vi "Render Delimiter.vi"(8 "Error In":errorcluster) -> (0 "Error Out":errorcluster)   [LabVIEW 2018, in "Tests.lvlib" / "Render.lvlib"]
uses:
  Render.lvlib
  src/Toolkit/Data/Map/Map.lvclass
  D:/Users/cfield/Code/Field R&D Services/Mustache/LabVIEW/trunk/src/Toolkit/Data/Abstract/Abstract.lvclass
  src/Toolkit/Low-Level/Support/Lex String.vi
  src/Toolkit/Data/Map/Support/From String Array.vi
  src/Toolkit/Low-Level/Support/Render to String.vi
  <vilib>/addons/_JKI Toolkits/Caraya/classes/Test/Test.lvclass
  <vilib>/addons/_JKI Toolkits/Caraya/classes/Assert/Assert.lvclass
  src/Toolkit/Toolkit.lvlib
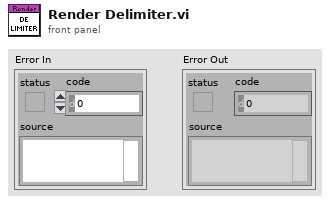
[diagram p1: front panel]
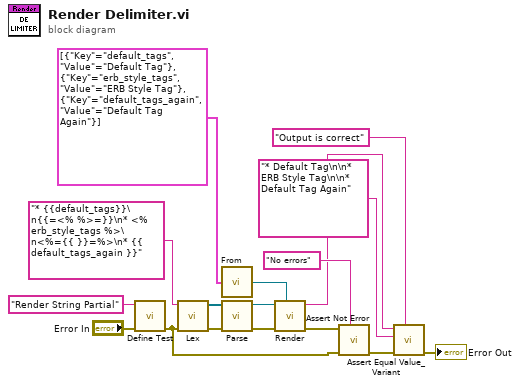
[diagram p0: block diagram]
diagram:
  n1 = call <vilib>:"Define Test.vi"("error in (no error)"="Error In", "Label (VI Title)"="Render String Partial") -> ("error out"=w5:errorcluster)  [unwired: 9 in]
  n2 = call-poly "Lex.vi"("Error In"=w5, "Input"="* {{default_tags}}\n{{=<% %>=}}\n* <% erb_style_tags %>\n<%={{ }}=%>\n* {{ default_tags_again }}" ("format string")) -> ("Error Out"=w7:errorcluster, "Tokens"=w8:refnum<class "Abstract.lvclass">[])  [unwired: 8 in]
  n3 = call-poly "From.vi"("Data"=cluster{"Key":string, "Value":string}[] [{"Key"="default_tags", "Value"="Default Tag"}, {"Key"="erb_style_tags", "Value"="ERB Style Tag"}, {"Key"="default_tags_again", "Value"="Default Tag Again"}]) -> ("Map"=w1:refnum<class "Map.lvclass">)  [unwired: 1 in]
  n4 = call "Parse.vi"("Error In"=w7, "Tokens"=w8) -> ("Error Out"=w9:errorcluster, "Abstract Syntax Tree"=w6:refnum<class "Root.lvclass">)  [unwired: 8 in]
  n5 = call-poly "Render.vi"("Data"=w1, "Error In"=w9, "Abstract Syntax Tree"=w6) -> ("Error Out"=w11:errorcluster, "Output"=w10:string)  [unwired: 7 in]
  n6 = call <vilib>:"Assert Not Error.vi"("Label"="No errors", "error in (no error)"=w5, "Not Error?"=w11) -> ("error out"=w14:errorcluster)  [unwired: 8 in]
  n7 = call <vilib>:"Assert Equal Value_Variant.vi"("Label"="Output is correct", "error in (no error)"=w14, "Y"="* Default Tag\n\n* ERB Style Tag\n\n* Default Tag Again", "X"=w10) -> ("error out"=→"Error Out":errorcluster)  [unwired: 7 in]
